vi "GetWebpageAndSave.vi"(8 "Error In":errorcluster, 9 "timeout (ms)":i32=1000, 10 "url":string, 11 "pathIn":path) -> (0 "error out":errorcluster, 3 "pathOut":path)   [LabVIEW 2015]
uses:
  <vilib>/httpClient/LabVIEWHTTPClient.lvlib
panel:
  out "headers":string
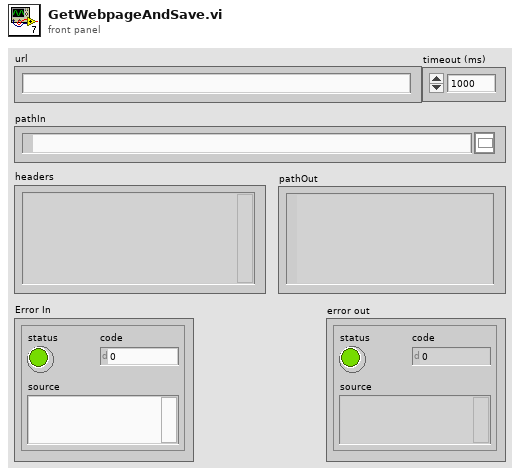
[diagram p1: front panel]
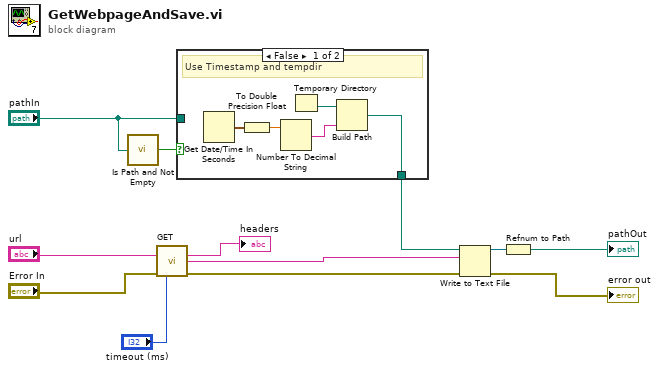
[diagram p0: block diagram]
diagram:
  n1 = call <vilib>:"Is Path and Not Empty.vi"("path"="pathIn") -> ("Is Path and Not Empty?"=w9:bool)  [unwired: 4 in]
  n2 = call <vilib>:"GET.vi"("url"="url", "error in (no error)"="Error In", "timeout (10000)"="timeout (ms)") -> ("headers"=→"headers":string, "body"=w4:string, "error out"=w11:errorcluster)  [unwired: 9 in, 1 out]
  n3 = case shown="False" w9 {
    tunnel: [w17 w18] -> w7
    tunnel: "pathIn" -> [_ w18]
    frame False {
      # "Use Timestamp and tempdir"
      n4 = Get Date/Time In Seconds() -> (seconds since 1Jan1904=w15:timestamp)
      n5 = To Double Precision Float(number=w15) -> (double precision float=w14:dbl)
      n6 = Number To Decimal String(number=w14) -> (decimal integer string=w13:string)  [unwired: 1 in]
      n7 = Temporary Directory() -> (w16:path)
      n8 = Build Path(base path=w16, name or relative path=w13) -> (appended path=w17:path)
    }
    frame True {
    }
  }
  n9 = Write to Text File(file (use dialog)=w7, text=w4, error in=w11) -> (refnum out=w5:refnum<file>, error out=→"error out":errorcluster)  [unwired: 1 in, 1 out]
  n10 = Refnum to Path(1:w5) -> (0:→"pathOut":path)
